vi "dfd_SCL_ARMABasicm_CU.vi"(8 "output valid":bool, 9 "global reset":bool, 11 "index":u16) -> (1 "control info":T1)   [LabVIEW 2017]
panel:
  in  "control info 2":T1
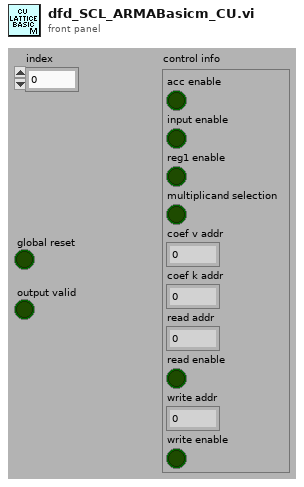
[diagram p1: front panel]
types:
  T1 = cluster{"acc enable":bool, "input enable":bool, "reg1 enable":bool, "multiplicand selection":bool, "coef v addr":u16, "coef k addr":u16, "read addr":u16, "read enable":bool, "write addr":u16, "write enable":bool}
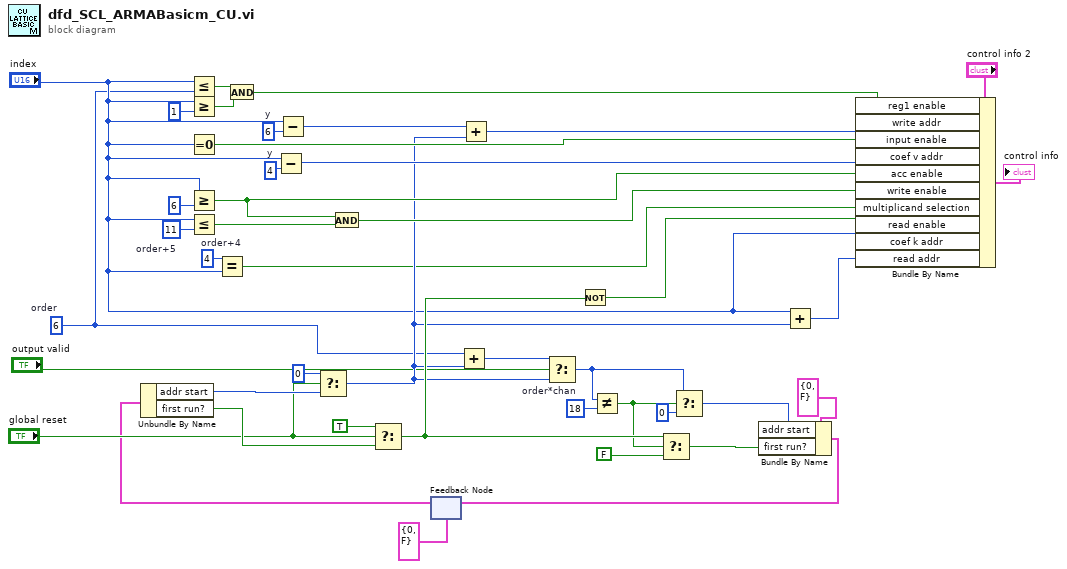
[diagram p0: block diagram]
diagram:
  w2 = u16 4  # order+4
  w22 = u16 11  # order+5
  w26 = u16 6  # y
  w27 = u16 4  # y
  w32 = u16 18  # order*chan
  w1 = u16 6  # order
  n1 = Less Or Equal?(x="index", y=w1) -> (x <= y?=w25:bool)
  n2 = Greater Or Equal?(x="index", y=u16 1) -> (x >= y?=w24:bool)
  n3 = Equal To 0?(x="index") -> (x = 0?=w18:bool)
  n4 = Greater Or Equal?(x="index", y=u16 6) -> (x >= y?=w16:bool)
  n5 = Less Or Equal?(x="index", y=w22) -> (x <= y?=w23:bool)
  n6 = Equal?(x=w2, y="index") -> (x = y?=w9:bool)
  n7 = And(x=w25, y=w24) -> (x .and. y?=w19:bool)
  n8 = Subtract(x="index", y=w27) -> (x-y=w17:u16)
  n9 = Subtract(x="index", y=w26) -> (x-y=w13:u16)
  n10 = And(x=w16, y=w23) -> (x .and. y?=w15:bool)
  n11 = feedback #1(cluster{"addr start":u16, "first run?":bool} {"addr start"=0, "first run?"=FALSE} ("states")) -> (w6:cluster{"addr start":u16, "first run?":bool})
  n12 = Unbundle By Name(w6) -> ("addr start"=w42:u16, "first run?"=w43:bool)
  n13 = Select(t=u16 0, s="global reset", f=w42) -> (s? t:f=w12:u16)
  n14 = Select(t=TRUE, s="global reset", f=w43) -> (s? t:f=w40:bool)
  n15 = Add(x=w1, y=w12) -> (x+y=w34:u16)
  n16 = Add(x=w13, y=w12) -> (x+y=w11:u16)
  n17 = Select(t=w34, s="output valid", f=w12) -> (s? t:f=w35:u16)
  n18 = Not(x=w40) -> (.not. x?=w8:bool)
  n19 = Not Equal?(x=w35, y=w32) -> (x != y?=w37:bool)
  n20 = Select(t=w40, s=w37, f=FALSE ("t")) -> (s? t:f=w41:bool)
  n21 = Select(t=w35, s=w37, f=u16 0) -> (s? t:f=w30:u16)
  n22 = Bundle By Name(cluster=cluster{"addr start":u16, "first run?":bool} {"addr start"=0, "first run?"=FALSE} ("states"), "addr start"=w30, "first run?"=w41) -> (w4:cluster{"addr start":u16, "first run?":bool})
  n23 = feedback-in #1(w4) -> ()
  n24 = Add(x="index", y=w12) -> (x+y=w14:u16)
  n25 = Bundle By Name(cluster="control info 2", "reg1 enable"=w19, "write addr"=w11, "input enable"=w18, "coef v addr"=w17, "acc enable"=w16, "write enable"=w15, "multiplicand selection"=w9, "read enable"=w8, "coef k addr"="index", "read addr"=w14) -> (→"control info":T1)
